vi "Temperature Controller.vi"(9 "Heater Range (0: Off)":u16(ring) items=["Off", "Low (0.5W)", "Med (5W)", "High (50W)"], 11 "Setpoint (0.0000)":dbl min=-273.0 max=300000.0 step=0.0001 format="%.4f") -> (18 "Loop 1\nHeater Output":dbl(slide) min=0.0 max=100.0 step=0.01 scale=0.0..100.0 scale format="%.1f")   [LabVIEW 2021]
doc: "This VI was designed to demonstrate typical usage of sub vi's containing the more common 331 functions.\n\nThis example configures the loop and setpoint of the instrument, allows for a delay, and then reads sensor and heater output data. The user is given the option of just reading data and not configuring the instrument."
uses:
  <instrlib>/Lake Shore Cryotronics 331/Lake Shore Cryotronics 331.lvlib
panel:
  out "Kelvin Reading":dbl min=0.0 max=1645.0 step=1e-05 format="%^.5e"
  in  "Input (0: A)":u16(ring) items=["A", "B"]
  in  "VISA resource name":refnum<visa-resource-name>
  # "(c) 2007-2009 Lake Shore Cryotronics Inc.  ALL RIGHTS RESERVED."
  # "331 Temperature Controller"
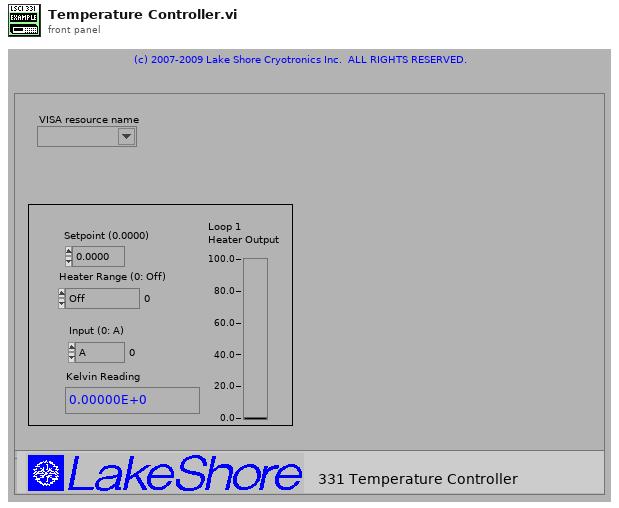
[diagram p1: front panel]
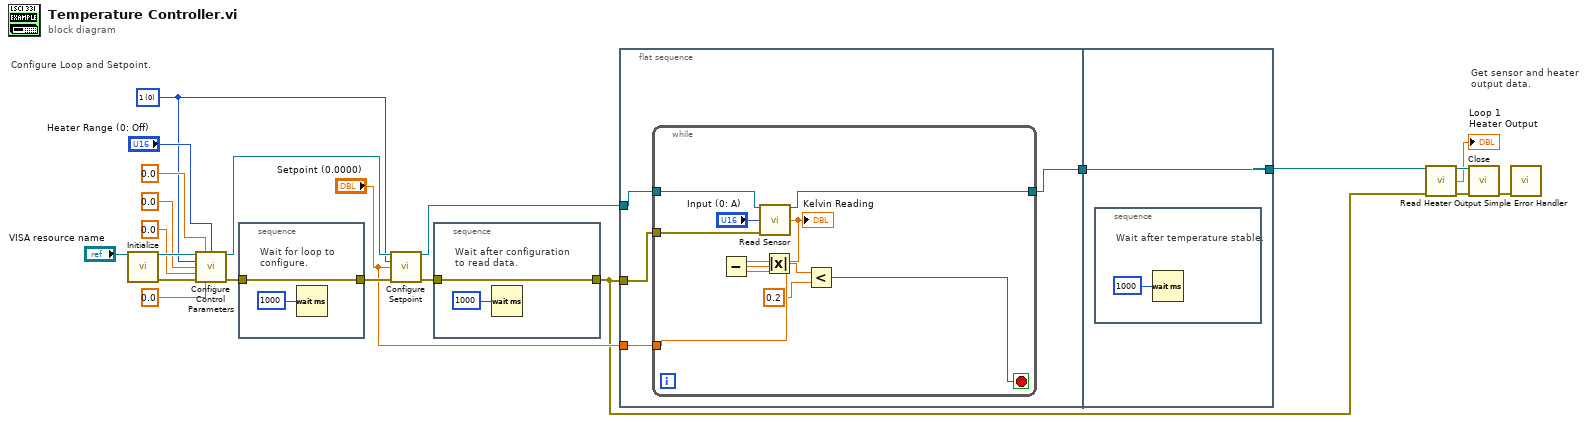
[diagram p0: block diagram]
diagram:
  w6 = u16 0 items=["1", "2"] ("Loop (0: 1)")
  # "Configure Loop and Setpoint."
  # "Get sensor and heater\noutput data."
  n1 = call <instrlib>:"Initialize.vi"("VISA resource name"="VISA resource name") -> ("VISA resource name out"=w21:refnum<visa-resource-name>, "error out"=w20:errorcluster)  [unwired: 13 in]
  n2 = call <instrlib>:"Configure Control Parameters.vi"("VISA resource name"=w21, "Manual Output (0.000 %)"=0.0 ("Manual Output (0.000)"), "Heater Range (0: Off)"="Heater Range (0: Off)", "Loop (0: 1)"=w6, "Gain (P) (0.0)"=0.0, "Reset (I) (0.0)"=0.0, "error in (no error)"=w20, "Rate (D) (0)"=0.0) -> ("VISA resource name out"=w7:refnum<visa-resource-name>, "error out"=w15:errorcluster)  [unwired: 6 in]
  n3 = stacked-sequence {
    tunnel: w15 -> [w23]
    tunnel: [w23] -> w9
    frame #0 {
      # "Wait for loop to \nconfigure."
      n4 = Wait (ms)(milliseconds to wait=u32 1000) -> ()  [unwired: 1 out]
    }
  }
  n5 = call <instrlib>:"Configure Setpoint.vi"("VISA resource name"=w7, "Loop (0: 1)"=w6, "Setpoint (0.0000)"="Setpoint (0.0000)", "error in (no error)"=w9) -> ("VISA resource name out"=w5:refnum<visa-resource-name>, "error out"=w8:errorcluster)  [unwired: 10 in]
  n6 = stacked-sequence {
    tunnel: w8 -> [w26]
    tunnel: [w26] -> w1
    frame #0 {
      # "Wait after configuration\nto read data."
      n7 = Wait (ms)(milliseconds to wait=1000) -> ()  [unwired: 1 out]
    }
  }
  n8 = flat-sequence {
    tunnel: w5 -> [w30]
    tunnel: w1 -> [w29]
    tunnel: "Setpoint (0.0000)" -> [w27]
    tunnel: [w28] -> w2
    tunnel: [w41] -> w4
    tunnel: w2 -> [w41]
    frame #0 {
      n9 = while {
        tunnel: w30 -> [w39]
        tunnel: w29 -> [w38]
        tunnel: [w37] -> w28
        tunnel: w27 -> [w36]
        stop <- w31 stop-if-true
        n10 = call <instrlib>:"Read Sensor.vi"("VISA resource name"=w39, "Input (0: A)"="Input (0: A)", "error in (no error)"=w38) -> ("VISA resource name out"=w37:refnum<visa-resource-name>, "Kelvin Reading"=w35:dbl)  [unwired: 8 in, 3 out]
        "Kelvin Reading" <- w35
        n11 = Subtract(x=w35, y=w36) -> (x-y=w34:dbl)
        n12 = Absolute Value(x=w34) -> (abs(x)=w33:dbl)
        n13 = Less?(x=w33, y=0.2) -> (x < y?=w31:bool)
      }
    }
    frame #1 {
      n14 = stacked-sequence {
        frame #0 {
          # "Wait after temperature stable."
          n15 = Wait (ms)(milliseconds to wait=1000) -> ()  [unwired: 1 out]
        }
      }
    }
  }
  n16 = call <instrlib>:"Read Heater Output.vi"("VISA resource name"=w4, "error in (no error)"=w1) -> ("VISA resource name out"=w17:refnum<visa-resource-name>, "Loop 1\nHeater Output"=→"Loop 1\nHeater Output":dbl, "error out"=w18:errorcluster)  [unwired: 11 in]
  n17 = call <instrlib>:"Close.vi"("VISA resource name"=w17, "error in (no error)"=w18) -> ("error out"=w22:errorcluster)  [unwired: 13 in]
  n18 = call <vilib>:"Simple Error Handler.vi"("error in (no error)"=w22) -> ()  [unwired: 4 in, 5 out]
